vi "GetQueue.vi"(8 "error in (no error)":errorcluster, 11 "Microscope in":refnum<class "Microscope.lvclass">) -> (0 "error out":errorcluster, 2 "Microscope events":refnum<queue>, 3 "Microscope out":refnum<class "Microscope.lvclass">)   [LabVIEW 2012, in "Microscope.lvclass"]
uses:
  classes/Microscope.lvclass
  typedefs/MicroscopeEvent.ctl
  classes/Microscope.lvclass/Microscope.ctl
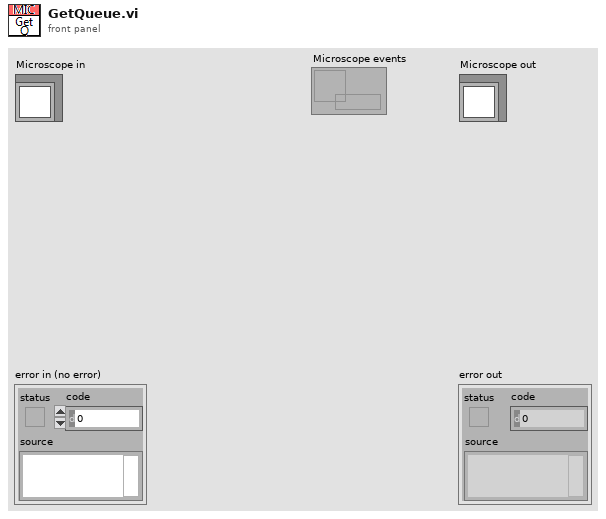
[diagram p1: front panel]
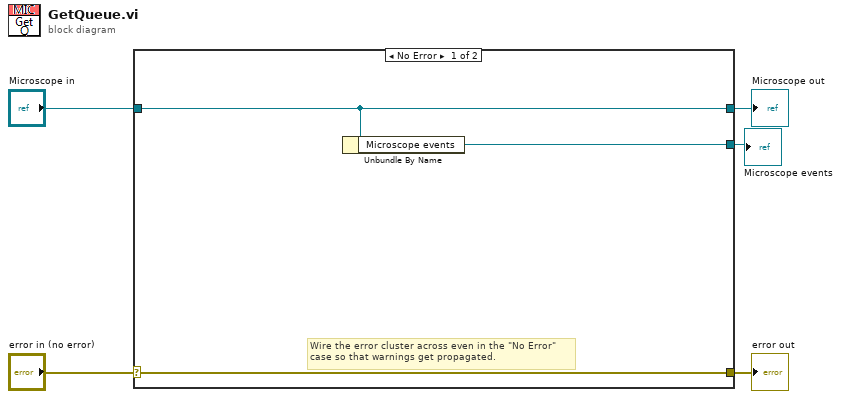
[diagram p0: block diagram]
diagram:
  n1 = case shown="No Error" "error in (no error)" {
    selector: "error in (no error)" -> [w8 w10]
    tunnel: [w8 w10] -> w4
    tunnel: [w7 w9] -> w2
    tunnel: "Microscope in" -> [w7 w9]
    tunnel: [w6 _] -> w1
    frame No Error {
      # "Wire the error cluster across even in the \"No Error\"\ncase so that warnings get propagated."
      n2 = Unbundle By Name(w7) -> ("Microscope events"=w6:refnum<queue>)
    }
    frame Error {
    }
  }
  "error out" <- w4
  "Microscope out" <- w2
  "Microscope events" <- w1
